vi "Processing_2DHistogram.vi"(0 "Log(G/G0)":dbl[](array[numeric]), 1 "Maximum Piezo / nm":dbl=3.0, 2 "Minimum Piezo / nm":dbl=-0.25, 3 "Number of Piezo / nm Bins (100) (100)":i32=700, 5 "Piezo / nm":dbl[](array[numeric]), 7 "Enable?":bool, 9 "Reset":bool, 11 "Error In":errorcluster, 12 "Maximum Log(G/G0)":dbl=0.5, 13 "Minimum Log(G/G0)":dbl=-6.0, 14 "Number of Log(G/G0) Bins (100)":i32=700) -> (4 "Histogram":i32[][](array[numeric]), 15 "Error Out":errorcluster)   [LabVIEW 2023]
panel:
  in  "Array":i32[][][](array[numeric])
  out "Waveform Graph":i32[][](graph)
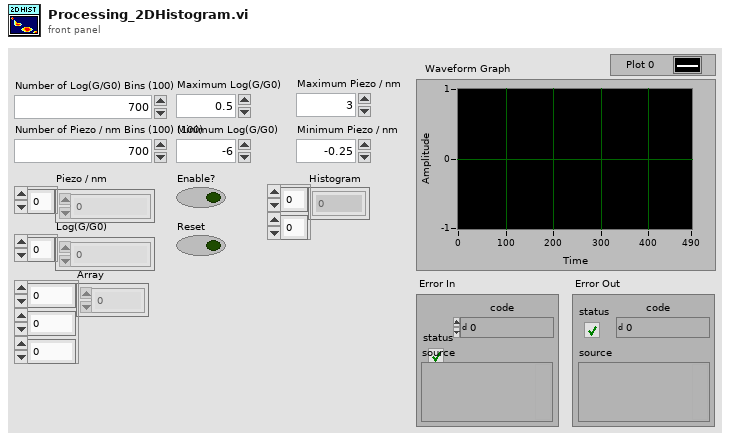
[diagram p1: front panel]
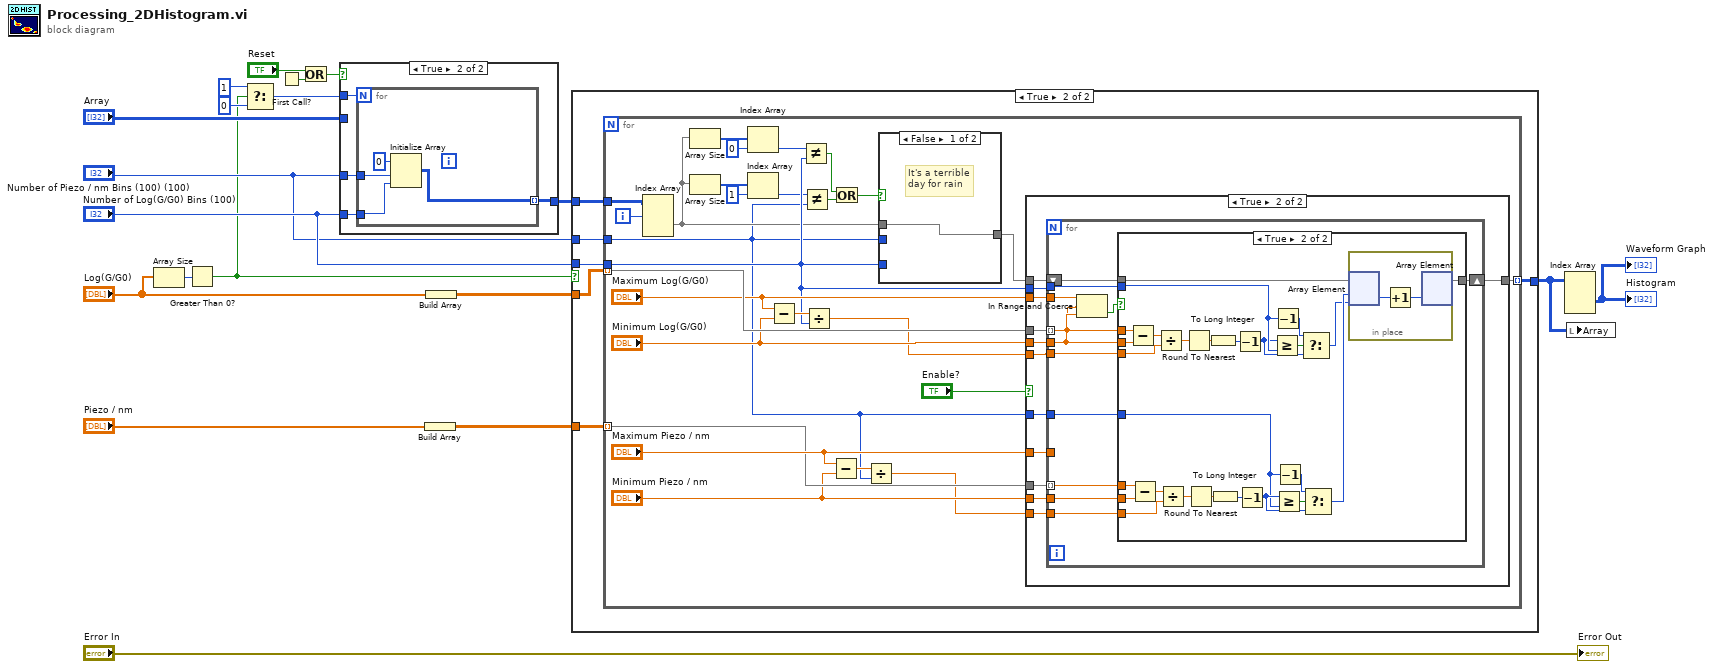
[diagram p0: block diagram]
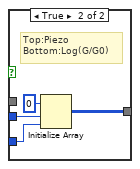
[diagram p5: hidden frame]
diagram:
  n1 = Array Size(array="Log(G/G0)") -> (size(s)=w5:i32)
  n2 = Greater Than 0?(x=w5) -> (x > 0?=w1:bool)
  n3 = Select(t=1, s=w1, f=0) -> (s? t:f=w2:i32)
  n4 = First Call?() -> (First Call?: T/F=w18:bool)
  n5 = Or(x="Reset", y=w18) -> (x .or. y?=w13:bool)
  n6 = case shown="True" w13 {
    tunnel: "Number of Log(G/G0) Bins (100)" -> [_ w24]
    tunnel: [w20 w23] -> w14
    tunnel: "Array" -> [w20 _]
    tunnel: w2 -> [_ w22]
    tunnel: "Number of Piezo / nm Bins (100) (100)" -> [_ w21]
    frame False {
      # "- isn't that becomming...\na race?\n\nAnd won't we be judged by\nhow we treat that race?"
    }
    frame True {
      n7 = for {
        N: w22 -> [_]
        tunnel: w24 -> [w26]
        tunnel: [w25] -> w23 mode=indexing
        tunnel: w21 -> [w27]
        n8 = Initialize Array(0, w27, w26) -> (w25:i32[][])
      }
    }
  }
  n9 = Build Array("Piezo / nm") -> (w11:dbl[][])
  n10 = Build Array("Log(G/G0)") -> (w15:dbl[][])
  n11 = case shown="True" w1 {
    tunnel: w14 -> [w29 w35]
    tunnel: w15 -> [_ w34]
    tunnel: [w29 w32] -> w7
    tunnel: "Number of Log(G/G0) Bins (100)" -> [_ w33]
    tunnel: w11 -> [_ w31]
    tunnel: "Number of Piezo / nm Bins (100) (100)" -> [_ w30]
    frame False {
      # "True. But it is not clear that a forseen doom long delayed\nis in all ways a lighter burden than one that comes soon. \nBut if I have understood your words thus far, you do not believe\nthat this difference was designed so in the beginning.\n\nYou were not at first doomed to swift death."
    }
    frame True {
      n12 = for {
        tunnel: w34 -> [w62] mode=indexing
        tunnel: w35 -> [w61]
        tunnel: w33 -> [w46]
        tunnel: [w55] -> w32 mode=indexing
        tunnel: w31 -> [w52] mode=indexing
        tunnel: w30 -> [w40]
        i -> [w36]
        n13 = Index Array(array=w61, index (dim 0)=w36) -> (element=w42:i32[][])  [unwired: 2 in]
        n14 = Array Size(array=w42) -> (size(s)=w49:i32[])
        n15 = Array Size(array=w42) -> (size(s)=w44:i32[])
        n16 = Index Array(array=w49, index=0) -> (element=w48:i32)
        n17 = Index Array(array=w44, index=1) -> (element=w41:i32)
        n18 = Subtract(x="Maximum Log(G/G0)", y="Minimum Log(G/G0)") -> (x-y=w57:dbl)
        n19 = Not Equal?(x=w48, y=w46) -> (x != y?=w38:bool)
        n20 = Not Equal?(x=w41, y=w40) -> (x != y?=w39:bool)
        n21 = Divide(x=w57, y=w46) -> (x/y=w56:dbl)
        n22 = Subtract(x="Maximum Piezo / nm", y="Minimum Piezo / nm") -> (x-y=w54:dbl)
        n23 = Or(x=w38, y=w39) -> (x .or. y?=w37:bool)
        n24 = Divide(x=w54, y=w40) -> (x/y=w50:dbl)
        n25 = case shown="False" w37 {
          tunnel: [w117 w118] -> w45
          tunnel: w42 -> [w117 _]
          tunnel: w46 -> [_ w119]
          tunnel: w40 -> [_ w120]
          frame False {
            # "It's a terrible\nday for rain"
          }
          frame True {
            # "Top:Piezo\nBottom:Log(G/G0)"
            n26 = Initialize Array(0, w120, w119) -> (w118:i32[][])
          }
        }
        n27 = case shown="True" "Enable?" {
          tunnel: "Minimum Log(G/G0)" -> [_ w75]
          tunnel: w62 -> [_ w74]
          tunnel: w45 -> [w63 w73]
          tunnel: [w63 w72] -> w55
          tunnel: "Maximum Log(G/G0)" -> [_ w71]
          tunnel: w56 -> [_ w70]
          tunnel: w46 -> [_ w69]
          tunnel: "Maximum Piezo / nm" -> [_ w68]
          tunnel: w52 -> [_ w67]
          tunnel: "Minimum Piezo / nm" -> [_ w66]
          tunnel: w50 -> [_ w65]
          tunnel: w40 -> [_ w64]
          frame False {
            # "Do you take me for a sponge, my Lord?\n\nAy, sir that soaks up the king’s countenance, his rewards, his authorities. \nBut such officers do the king best service in the end. He keeps them, like an ape,\nin the corner of his jaw, first mouthed to be last swallowed. When he needs\nwhat you have gleaned, it is but squeezing you and, sponge,\nyou shall be dry again.\n\nI understand you not, my lord.\n\nI am glad of it. A knavish speech sleeps in a foolish ear."
          }
          frame True {
            n28 = for {
              tunnel: w74 -> [w82] mode=indexing
              tunnel: w75 -> [w83]
              tunnel: w70 -> [w87]
              shift-right: [w85] -> w72
              shift-left: w73 -> [w86]
              tunnel: w71 -> [w84]
              tunnel: w69 -> [w81]
              tunnel: w68 -> [_]
              tunnel: w67 -> [w79] mode=indexing
              tunnel: w66 -> [w78]
              tunnel: w65 -> [w77]
              tunnel: w64 -> [w76]
              n29 = In Range and Coerce(upper limit=w84, x=w82, lower limit=w83) -> (In Range?=w80:bool)  [unwired: 1 out]
              n30 = case shown="True" w80 {
                tunnel: w87 -> [_ w113]
                tunnel: w86 -> [w88 w110]
                tunnel: [w88 w109] -> w85
                tunnel: w83 -> [_ w108]
                tunnel: w82 -> [_ w107]
                tunnel: w81 -> [_ w105]
                tunnel: w79 -> [_ w94]
                tunnel: w78 -> [_ w93]
                tunnel: w77 -> [_ w92]
                tunnel: w76 -> [_ w91]
                frame False {
                  # "I'm looking for a great warrior...\n\nWars not make one great."
                }
                frame True {
                  n31 = Subtract(x=w107, y=w108) -> (x-y=w114:dbl)
                  n32 = Subtract(x=w94, y=w93) -> (x-y=w101:dbl)
                  n33 = Divide(x=w114, y=w113) -> (x/y=w112:dbl)
                  n34 = Divide(x=w101, y=w92) -> (x/y=w100:dbl)
                  n35 = Round To Nearest(number=w112) -> (nearest integer value=w111:dbl)
                  n36 = Round To Nearest(number=w100) -> (nearest integer value=w99:dbl)
                  n37 = To Long Integer(number=w111) -> (32bit integer=w103:i32)
                  n38 = To Long Integer(number=w99) -> (32bit integer=w96:i32)
                  n39 = Decrement(x=w103) -> (x-1=w102:i32)
                  n40 = Decrement(x=w96) -> (x-1=w95:i32)
                  n41 = Greater Or Equal?(x=w102, y=w105) -> (x >= y?=w106:bool)
                  n42 = Decrement(x=w105) -> (x-1=w104:i32)
                  n43 = Greater Or Equal?(x=w95, y=w91) -> (x >= y?=w98:bool)
                  n44 = Decrement(x=w91) -> (x-1=w97:i32)
                  n45 = Select(t=w104, s=w106, f=w102) -> (s? t:f=w89:i32)
                  n46 = Select(t=w97, s=w98, f=w95) -> (s? t:f=w90:i32)
                  n47 = in-place {
                    n48 = in-place-array #1(w110, w90, w89) -> (w115:i32)
                    n49 = Increment(x=w115) -> (x+1=w116:i32)
                    n50 = in-place-array #1(w116) -> (w109:i32[][])  [unwired: 2 out]
                  }
                }
              }
            }
          }
        }
      }
    }
  }
  n51 = Index Array(array=w7) -> (element=→"Waveform Graph" →"Histogram":i32[][])  [unwired: 3 in]
  n52 = local write "Array"(w7) -> ()
  "Error Out" <- "Error In"
